vi "CIF Template UI.vi"() -> ()   [LabVIEW 2021, in "CIF Template UI.lvlib"]
uses:
  CIF Template UI.lvlib
  CIF-LVCore/src/CIFUI/Typedef/Run Listen Button.ctl
  CIF-LVCore/src/CIFUI/Typedef/Core UI References.ctl
  CIF-LVCore/src/CIFUI/CIF_UI.lvclass/CIF_UI.ctl
  CIF-LVCore/src/CIFUI/Utilities/Get Human Readable Error.vi
  CIF-LVCore/src/CIFUI/UI Element Update/Empty Tree by Reference.vi
  CIF-LVCore/src/CIFUI/UI Element Update/Empty Table by Reference.vi
  CIF-LVCore/src/CIFUI/UI Element Update/Initialize Manager Tab by Reference.vi
  <vilib>/CIF Foundation/CIF Utilities/Errors/Human Readable Error Message.vi
  CIF-LVCore/src/CIFUI/CIF_UI.lvclass
  Grpc/Template_wrapper/TemplateWrapper.lvlib
  <vilib>/Utility/LVLibp/NI_PackedLibraryUtility.lvlib
panel:
  in  "Session Id":u64
  in  "EXIT":bool
  in  "Address with Port":string="192.168.1.160:12345"
  in  "Clear Local Error":bool
  out "Connected":bool
  in  "Unload":bool
  in  "Refresh Button":bool
  in  "Run Listen":T1
  in  "Connection":bool
  out "Local Error":string
  in  "Plugin Status":string[][](table)
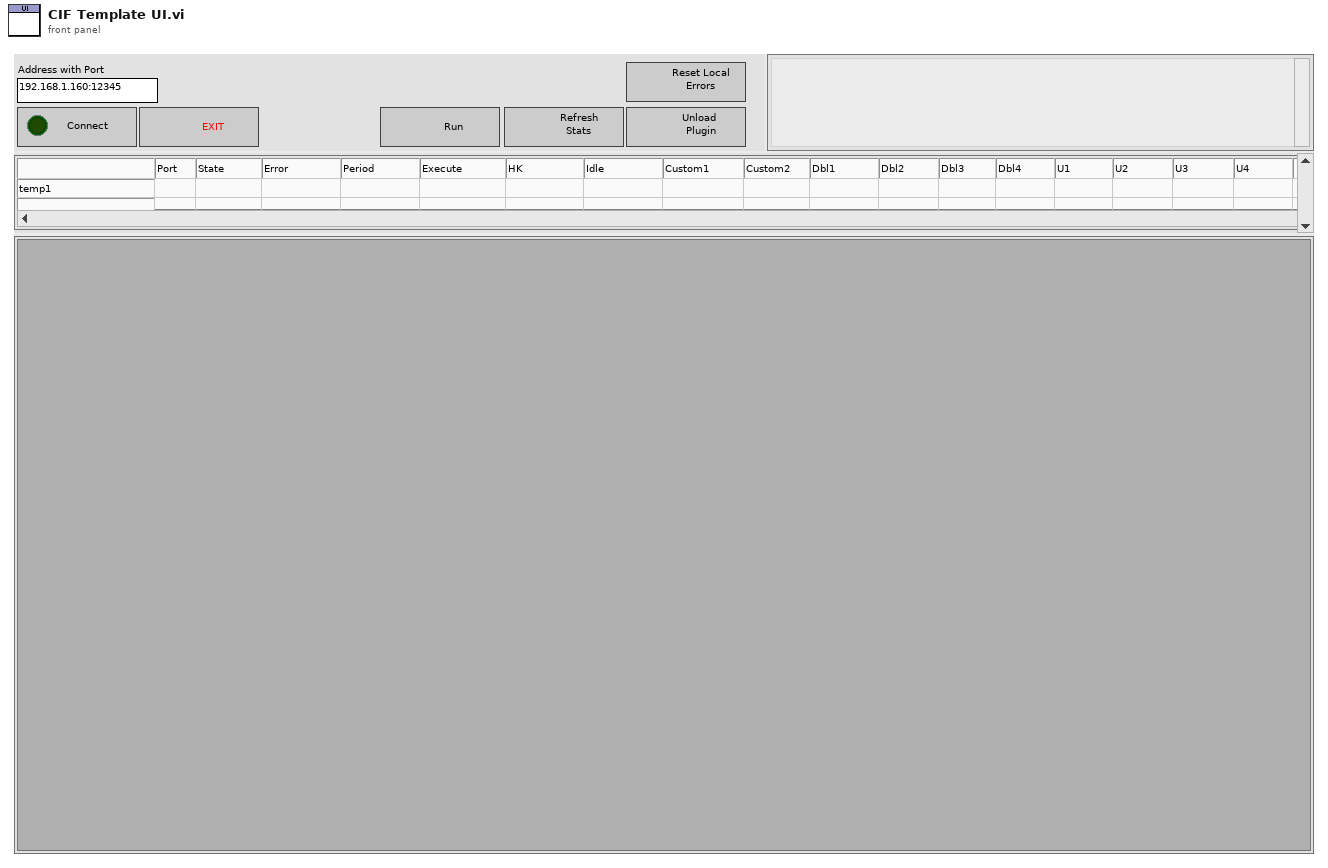
[diagram p1: front panel]
types:
  T1 = typedef "CIF_UI.lvclass/Run Listen Button.ctl" = bool
  T2 = typedef "CIF_UI.lvclass/Core UI References.ctl" = cluster{"Discovered Plugins":refnum<vi>, "Discovered Plugins Valid":bool, "Loaded Plugins":refnum<vi>, "Loaded Plugins Valid":bool, "Publisher Channels":refnum<vi>, "Publisher Channels Valid":bool, "Subscriber Channels":refnum<vi>, "Subscriber Channels Valid":bool, "Plugin Status":refnum<vi>, "Plugin Status Valid":bool, "Channel Connection":refnum<vi>, "Channel Connection Valid":bool, "New Plugin Load":refnum<vi>, "New Plugin Load Valid":bool, "Errors":refnum<vi>, "Errors Valid":bool, "Plugin to Abort":refnum<vi>, "Plugin to Abort Valid":bool, "Connection":refnum<vi>, "Connection Valid":bool, "Exit":refnum<vi>, "Exit Valid":bool, "Run Listen":refnum<vi>, "Run Listen Valid":bool, "CIF Manager Tab":refnum<vi>, "Manger Tab Valid":bool, "Clear Local Error":refnum<vi>, "Clear Local Error Valid":bool, "Local Error":refnum<vi>, "Local Error Valid":bool, "System Errors":refnum<vi>, "System Errors Valid":bool, "Plugin Selection":refnum<vi>, "Plugin Selection Valid":bool}
  T3 = typedef "InstrumentStudio Plugin SDK.lvlib/Event Registration Refnum.ctl" = refnum<event-registration>
  T4 = cluster{"Event Refnum":T3, "Event Registration Refnum":refnum<event-registration>}
  T5 = typedef "grpc-lvsupport-release.lvlib/grpcId.ctl" = u64
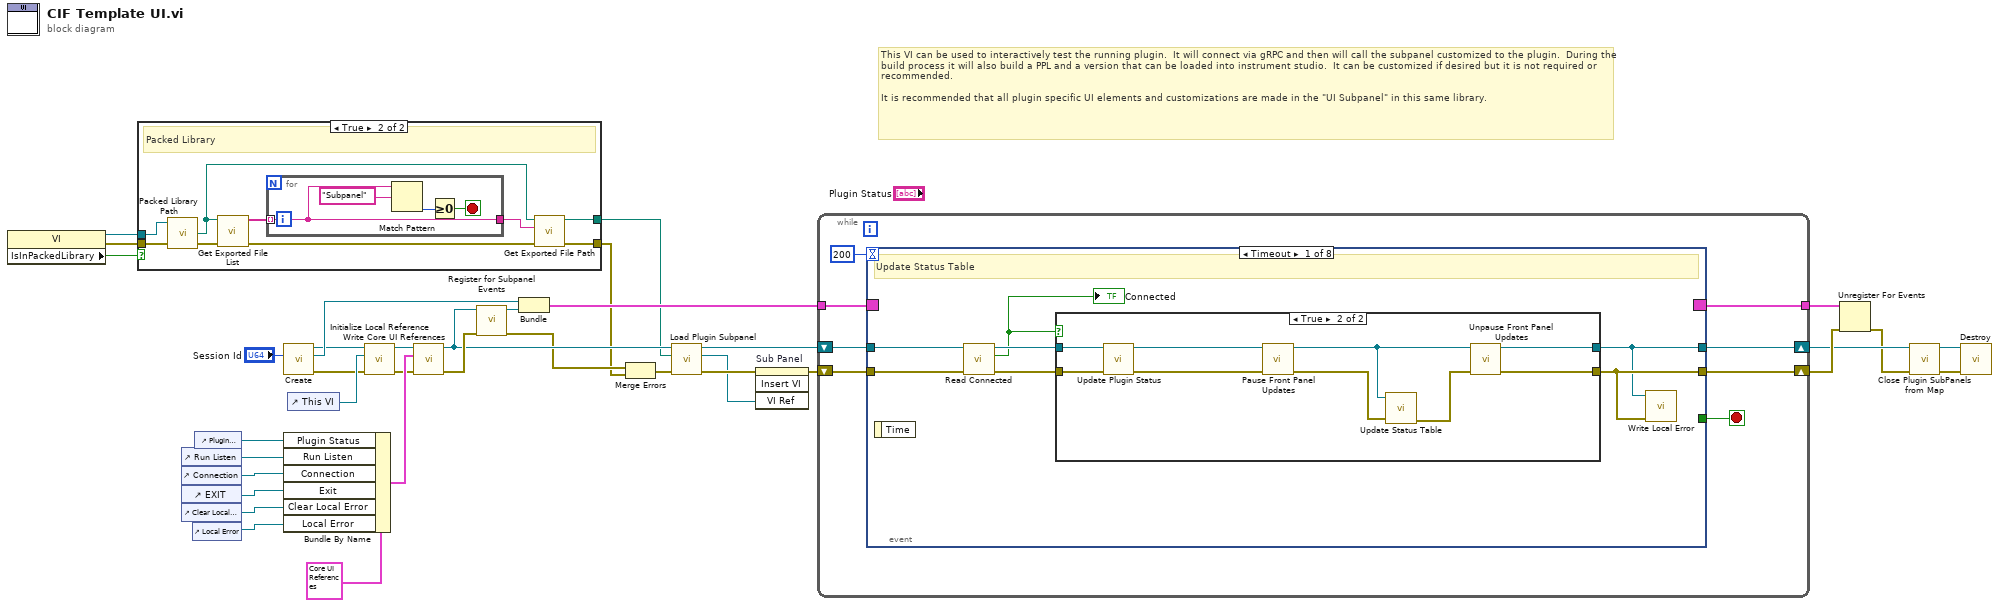
[diagram p0: block diagram]
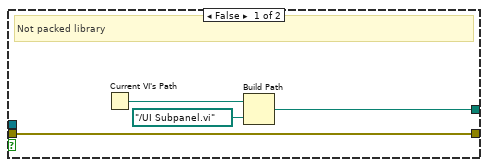
[diagram p2: hidden frame]
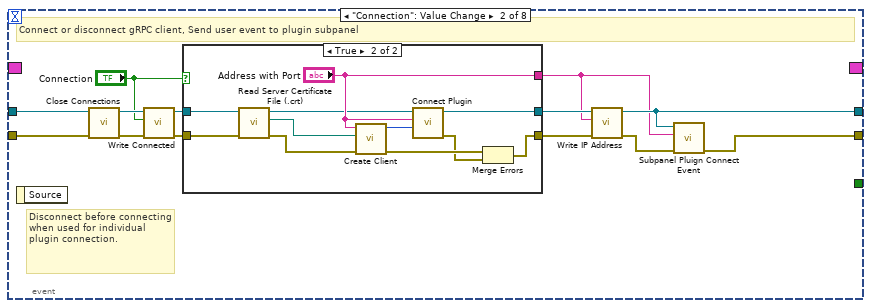
[diagram p4: hidden frame]
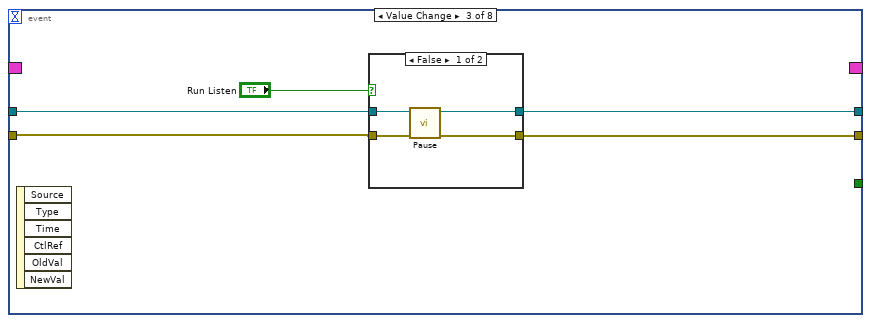
[diagram p6: hidden frame]
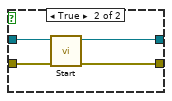
[diagram p7: hidden frame]
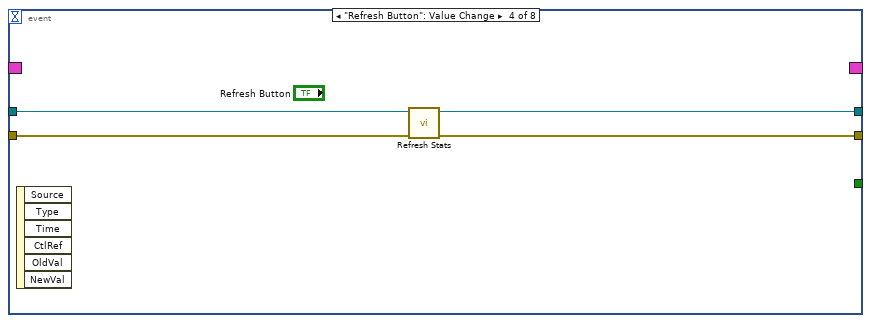
[diagram p8: hidden frame]
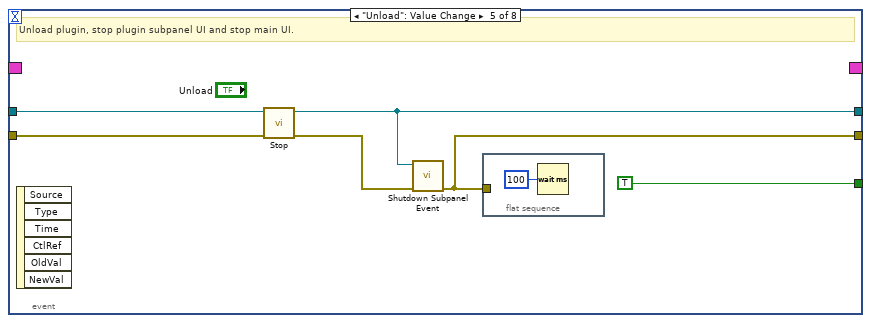
[diagram p9: hidden frame]
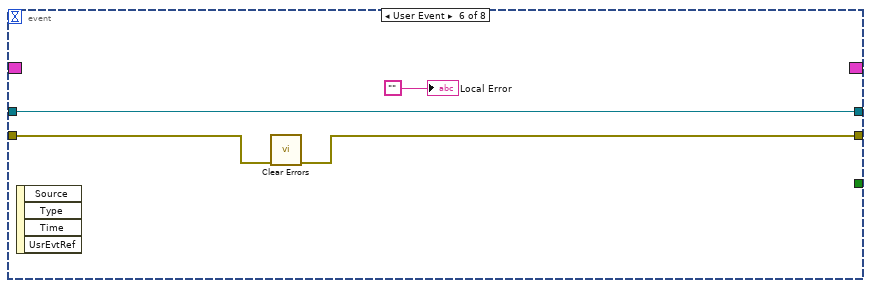
[diagram p10: hidden frame]
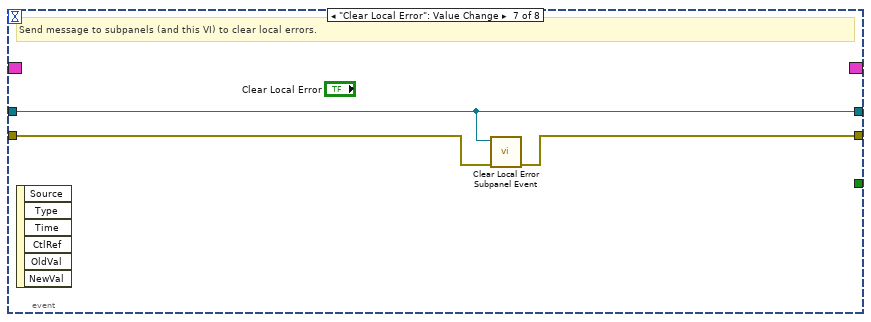
[diagram p11: hidden frame]
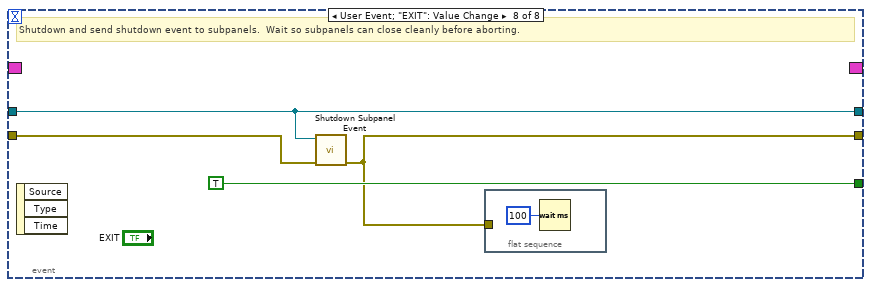
[diagram p12: hidden frame]
diagram:
  # "This VI can be used to interactively test the running plugin.  It will connect via gRPC and then will call the subpanel customized to the plugin.  During the build process it will also build a PPL and a version that can be loaded into instrument studio.  It can be customized if desired but it is not required or recommended.  \n\nIt is recommended that all plugin specific UI elements and customizations are made in the \"UI Subpanel\" in this same library."
  n1 = property class="VI"() -> (reference out=w7:refnum<vi>, error out=w6:errorcluster, "IsInPackedLibrary"=w8:bool)  [unwired: 2 in]
  n2 = case shown="True" w8 {
    tunnel: w7 -> [_ w49]
    tunnel: w6 -> [w37 w48]
    tunnel: [w40 w42] -> w5
    tunnel: [w37 w41] -> w2
    frame False {
      # "Not packed library"
      n3 = Current VI's Path() -> (path=w39:path)
      n4 = Build Path(base path=w39, name or relative path=path "../UI Subpanel.vi" ("Path")) -> (appended path=w40:path)
    }
    frame True {
      # "Packed Library"
      n5 = call <vilib>:"Packed Library Path.vi"("error in (no error)"=w48, "vi reference"=w49) -> ("error out"=w43:errorcluster, "packed library path"=w44:path)  [unwired: 1 in, 1 out]
      n6 = call <vilib>:"Get Exported File List.vi"("error in (no error)"=w43, "packed library path"=w44) -> ("error out"=w46:errorcluster, "qualified names"=w45:string[])  [unwired: 7 in, 1 out]
      n7 = for {
        tunnel: w45 -> [w50] mode=indexing
        tunnel: [w50] -> w47
        stop <- w52 stop-if-true
        n8 = Match Pattern(string=w50, regular expression="Subpanel") -> (offset past match=w53:i32)  [unwired: 1 in, 3 out]
        n9 = Greater Or Equal To 0?(x=w53) -> (x >= 0?=w52:bool)
      }
      n10 = call <vilib>:"Get Exported File Path.vi"("error in (no error)"=w46, "qualified name"=w47, "packed library path"=w44) -> ("error out"=w41:errorcluster, "path"=w42:path)  [unwired: 7 in]
    }
  }
  n11 = control-ref of="Run Listen"() -> (w30:refnum<vi>)
  n12 = control-ref of="Connection"() -> (w27:refnum<vi>)
  n13 = control-ref of="EXIT"() -> (w26:refnum<vi>)
  n14 = control-ref of="Clear Local Error"() -> (w25:refnum<vi>)
  n15 = control-ref of="Local Error"() -> (w24:refnum<vi>)
  n16 = control-ref of="Plugin Status"() -> (w34:refnum<vi>)
  n17 = call "Create.vi"("Session Id"="Session Id") -> ("error out"=w21:errorcluster, "Event Refnum"=w28:T3, "CIF_UI out"=w22:refnum<class "CIF_UI.lvclass">)  [unwired: 8 in]
  n18 = Bundle By Name(cluster=T2 {"Discovered Plugins"=refnum, "Discovered Plugins Valid"=FALSE, "Loaded Plugins"=refnum, "Loaded Plugins Valid"=FALSE, "Publisher Channels"=refnum, "Publisher Channels Valid"=FALSE, "Subscriber Channels"=refnum, "Subscriber Channels Valid"=FALSE, "Plugin Status"=refnum, "Plugin Status Valid"=FALSE, "Channel Connection"=refnum, "Channel Connection Valid"=FALSE, "New Plugin Load"=refnum, "New Plugin Load Valid"=FALSE, "Errors"=refnum, "Errors Valid"=FALSE, "Plugin to Abort"=refnum, "Plugin to Abort Valid"=FALSE, "Connection"=refnum, "Connection Valid"=FALSE, "Exit"=refnum, "Exit Valid"=FALSE, "Run Listen"=refnum, "Run Listen Valid"=FALSE, "CIF Manager Tab"=refnum, "Manger Tab Valid"=FALSE, "Clear Local Error"=refnum, "Clear Local Error Valid"=FALSE, "Local Error"=refnum, "Local Error Valid"=FALSE, "System Errors"=refnum, "System Errors Valid"=FALSE, "Plugin Selection"=refnum, "Plugin Selection Valid"=FALSE} ("UI References"), "Plugin Status"=w34, "Run Listen"=w30, "Connection"=w27, "Exit"=w26, "Clear Local Error"=w25, "Local Error"=w24) -> (w35:T2)
  n19 = control-ref of="This VI"() -> (w33:refnum<vi>)
  n20 = call "Initialize Local Reference.vi"("error in (no error)"=w21, "This VI"=w33, "CIF_UI in"=w22) -> ("error out"=w31:errorcluster, "CIF_UI out"=w32:refnum<class "CIF_UI.lvclass">)  [unwired: 7 in]
  n21 = call "Write Core UI References.vi"("error in (no error)"=w31, "UI References"=w35, "CIF_UI in"=w32) -> ("error out"=w20:errorcluster, "CIF_UI out"=w17:refnum<class "CIF_UI.lvclass">)  [unwired: 7 in]
  n22 = call "Register for Subpanel Events.vi"("error in (no error)"=w20, "CIF_UI in"=w17) -> ("error out"=w4:errorcluster, "Event Registration Refnum"=w29:refnum<event-registration>)  [unwired: 8 in]
  n23 = Bundle("Event Refnum"=w28, "Event Registration Refnum"=w29) -> (w23:T4)  [unwired: 1 in]
  n24 = Merge Errors(w4, w2) -> (w3:errorcluster)
  n25 = call "Load Plugin Subpanel.vi"("error in (no error)"=w3, "Path"=w5, "CIF_UI in"=w17) -> ("error out"=w15:errorcluster, "VI Reference"=w13:refnum<vi>, "CIF_UI out"=w16:refnum<class "CIF_UI.lvclass">)  [unwired: 6 in]
  n26 = invoke on="Sub Panel" class="SubPnl" method="Insert VI"(error in=w15, "VI Ref"=w13) -> (error out=w14:errorcluster)  [unwired: 2 in, 3 out]
  n27 = while {
    shift-right: [w56] -> w12
    shift-left: w16 -> [w59]
    shift-right: [w57] -> w18
    shift-left: w14 -> [w58]
    tunnel: w23 -> [w55]
    tunnel: [w54] -> w19
    stop <- w60 stop-if-true
    n28 = event shown="[0] Timeout" {
      selector: w55 -> [_ _ _ _ _ _ _ _]
      dyn-events: [_ _ _ _ _ _ _ _] -> w54
      timeout: 200 -> [_ _ _ _ _ _ _ _]
      tunnel: [_ _ _ _ TRUE _ _ TRUE] -> w60
      tunnel: w59 -> [w66 w91 w110 w122 w128 w131 w134 w139]
      tunnel: w58 -> [w65 w92 w108 w120 w127 w133 w136 w138]
      tunnel: [w63 w80 w106 w119 w124 w132 w135 w137] -> w57
      tunnel: [w62 w83 w107 w121 w125 w131 w134 w139] -> w56
      event Timeout {
        # "Update Status Table"
        n29 = event-data() -> ()  [unwired: 1 in, 1 out]
        n30 = call "Read Connected.vi"("error in (no error)"=w65, "CIF_UI in"=w66) -> ("error out"=w67:errorcluster, "Connected"=w64:bool, "CIF_UI out"=w68:refnum<class "CIF_UI.lvclass">)  [unwired: 7 in]
        "Connected" <- w64
        n31 = case shown="True" w64 {
          tunnel: w67 -> [w69 w77]
          tunnel: [w69 w79] -> w63
          tunnel: w68 -> [w70 w76]
          tunnel: [w70 w78] -> w62
          frame False {
          }
          frame True {
            n32 = call "Update Plugin Status.vi"("error in (no error)"=w77, "CIF_UI in"=w76) -> ("error out"=w71:errorcluster, "CIF_UI out"=w75:refnum<class "CIF_UI.lvclass">)  [unwired: 8 in]
            n33 = call "Pause Front Panel Updates.vi"("error in (no error)"=w71, "CIF_UI in"=w75) -> ("error out"=w74:errorcluster, "CIF_UI out"=w73:refnum<class "CIF_UI.lvclass">)  [unwired: 8 in]
            n34 = call "Update Status Table.vi"("error in (no error)"=w74, "CIFManager_UI in"=w73) -> ("error out"=w72:errorcluster)  [unwired: 9 in]
            n35 = call "Unpause Front Panel Updates.vi"("error in (no error)"=w72, "CIF_UI in"=w73) -> ("error out"=w79:errorcluster, "CIF_UI out"=w78:refnum<class "CIF_UI.lvclass">)  [unwired: 8 in]
          }
        }
        n36 = call "Write Local Error.vi"("error in (no error)"=w63, "CIF_UI in"=w62) -> ()  [unwired: 9 in, 1 out]
      }
      event "Connection": Value Change {
        # "Disconnect before connecting when used for individual plugin connection."
        # "Connect or disconnect gRPC client, Send user event to plugin subpanel"
        n37 = event-data() -> ()  [unwired: 1 in, 1 out]
        n38 = call "Close Connections.vi"("error in (no error)"=w92, "CIF_UI in"=w91) -> ("error out"=w89:errorcluster, "CIF_UI out"=w90:refnum<class "CIF_UI.lvclass">)  [unwired: 8 in]
        n39 = call "Write Connected.vi"("error in (no error)"=w89, "Connected"="Connection", "CIF_UI in"=w90) -> ("error out"=w86:errorcluster, "CIF_UI out"=w88:refnum<class "CIF_UI.lvclass">)  [unwired: 7 in]
        n40 = case shown="True" "Connection" {
          tunnel: [w94 w101] -> w85
          tunnel: [w93 w105] -> w84
          tunnel: w86 -> [w93 w98]
          tunnel: w88 -> [w94 w99]
          tunnel: [_ "Address with Port"] -> w81
          frame False {
          }
          frame True {
            n41 = call "Read Server Certificate File (.crt).vi"("error in (no error)"=w98, "CIF_UI in"=w99) -> ("error out"=w97:errorcluster, "Server Certificate File (.crt)"=w96:path, "CIF_UI out"=w95:refnum<class "CIF_UI.lvclass">)  [unwired: 7 in]
            n42 = call "Create Client.vi"("error in"=w97, "Server Certificate File (.crt)"=w96, "address"="Address with Port") -> ("error out"=w103:errorcluster, "gRPC ID Out"=w104:T5)  [unwired: 7 in]
            n43 = call "Connect Plugin.vi"("gRPC ID"=w104, "Address"="Address with Port", "CIF_UI in"=w95) -> ("error out"=w102:errorcluster, "CIF_UI out"=w101:refnum<class "CIF_UI.lvclass">)  [unwired: 7 in]
            n44 = Merge Errors(w103, w102) -> (w105:errorcluster)
          }
        }
        n45 = call "Write IP Address.vi"("error in (no error)"=w84, "IP Address"=w81, "CIF_UI in"=w85) -> ("error out"=w82:errorcluster, "CIF_UI out"=w83:refnum<class "CIF_UI.lvclass">)  [unwired: 7 in]
        n46 = call "Subpanel Pluign Connect Event.vi"("error in (no error)"=w82, "Address and Port"=w81, "CIF_UI in"=w83) -> ("error out"=w80:errorcluster)  [unwired: 8 in]
      }
      event Value Change {
        n47 = event-data() -> ()  [unwired: 1 in, 6 out]
        n48 = case shown="False" "Run Listen" {
          tunnel: w108 -> [w114 w118]
          tunnel: w110 -> [w113 w117]
          tunnel: [w111 w116] -> w107
          tunnel: [w112 w115] -> w106
          frame False {
            n49 = call "Pause.vi"("error in (no error)"=w114, "CIF_Plugin_UI in"=w113) -> ("error out"=w112:errorcluster, "CIF_Plugin_UI out"=w111:refnum<class "CIF_UI.lvclass">)  [unwired: 7 in, 1 out]
          }
          frame True {
            n50 = call "Start.vi"("error in (no error)"=w118, "CIF_Plugin_UI in"=w117) -> ("error out"=w115:errorcluster, "CIF_Plugin_UI out"=w116:refnum<class "CIF_UI.lvclass">)  [unwired: 7 in, 1 out]
          }
        }
      }
      event "Refresh Button": Value Change {
        n51 = event-data() -> ()  [unwired: 1 in, 6 out]
        n52 = call "Refresh Stats.vi"("error in (no error)"=w120, "CIF_Plugin_UI in"=w122) -> ("error out"=w119:errorcluster, "CIF_Plugin_UI out"=w121:refnum<class "CIF_UI.lvclass">)  [unwired: 7 in, 1 out]
      }
      event "Unload": Value Change {
        # "Unload plugin, stop plugin subpanel UI and stop main UI."
        n53 = event-data() -> ()  [unwired: 1 in, 6 out]
        n54 = call "Stop.vi"("error in (no error)"=w127, "CIF_Plugin_UI in"=w128) -> ("error out"=w126:errorcluster, "CIF_Plugin_UI out"=w125:refnum<class "CIF_UI.lvclass">)  [unwired: 7 in, 1 out]
        n55 = call "Shutdown Subpanel Event.vi"("error in (no error)"=w126, "CIF_UI in"=w125) -> ("error out"=w124:errorcluster)  [unwired: 9 in]
        n56 = flat-sequence {
          tunnel: w124 -> [_]
          frame #0 {
            n57 = Wait (ms)(milliseconds to wait=u32 100) -> ()  [unwired: 1 out]
          }
        }
      }
      event User Event {
        n58 = event-data() -> ()  [unwired: 1 in, 4 out]
        n59 = call <vilib>:"Clear Errors.vi"("error in (no error)"=w133) -> ("error out"=w132:errorcluster)  [unwired: 5 in, 1 out]
        "Local Error" <- ""
      }
      event "Clear Local Error": Value Change {
        # "Send message to subpanels (and this VI) to clear local errors."
        n60 = event-data() -> ()  [unwired: 1 in, 6 out]
        n61 = call "Clear Local Error Subpanel Event.vi"("error in (no error)"=w136, "CIF_UI in"=w134) -> ("error out"=w135:errorcluster)  [unwired: 9 in]
      }
      event User Event; "EXIT": Value Change {
        # "Shutdown and send shutdown event to subpanels.  Wait so subpanels can close cleanly before aborting."
        n62 = event-data() -> ()  [unwired: 1 in, 3 out]
        n63 = call "Shutdown Subpanel Event.vi"("error in (no error)"=w138, "CIF_UI in"=w139) -> ("error out"=w137:errorcluster)  [unwired: 9 in]
        n64 = flat-sequence {
          tunnel: w137 -> [_]
          frame #0 {
            n65 = Wait (ms)(milliseconds to wait=u32 100) -> ()  [unwired: 1 out]
          }
        }
      }
    }
  }
  n66 = Unregister For Events(event registration refnum=w19, error in=w18) -> (error out=w11:errorcluster)
  n67 = call "Close Plugin SubPanels from Map.vi"("error in (no error)"=w11, "CIF_UI in"=w12) -> ("error out"=w10:errorcluster, "CIF_UI out"=w9:refnum<class "CIF_UI.lvclass">)  [unwired: 8 in]
  n68 = call "Destroy.vi"("error in (no error)"=w10, "CIF_UI in"=w9) -> ()  [unwired: 8 in, 2 out]
